vi "mbug_2820_single_acq.vi"() -> ()   [LabVIEW 2014]
doc: "This example shows how to acquire a power measurement using the VIs of the driver."
uses:
  <instrlib>/MBUG-2820/Private/Open_serial.vi
  <instrlib>/MBUG-2820/MBUG-2820.lvlib
panel:
  out "Rel. humidity (%)":dbl
  in  "Device serial (0: any)":u32 max=999999
  out "Temperature (°C)":dbl
  # "MBUG-2820 single acquisition example"
  # "Choose a device serial to open. ( 0: open the first available device.)"
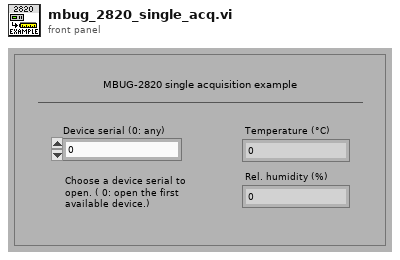
[diagram p1: front panel]
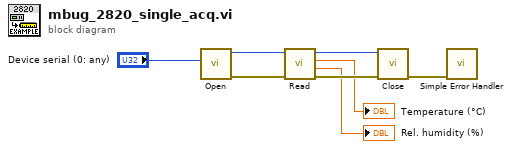
[diagram p0: block diagram]
diagram:
  n1 = call-poly <instrlib>:"Open.vi"("Device serial (0=any)"="Device serial (0: any)") -> ("error out"=w1:errorcluster, "Device handle"=w2:u32)  [unwired: 5 in]
  n2 = call <instrlib>:"Read.vi"("error in (no error)"=w1, "Device handle in"=w2) -> ("error out"=w7:errorcluster, "Rel. humidity (%)"=→"Rel. humidity (%)":dbl, "Temperature (°C)"=→"Temperature (°C)":dbl, "Device handle out"=w8:u32)  [unwired: 2 in]
  n3 = call <instrlib>:"Close.vi"("error in (no error)"=w7, "Device handle"=w8) -> ("error out"=w6:errorcluster)  [unwired: 5 in]
  n4 = call <vilib>:"Simple Error Handler.vi"("error in (no error)"=w6) -> ()  [unwired: 4 in, 5 out]
